vi "Denoise - 1D Real Signal.vi"() -> ()   [LabVIEW 2023]
doc: "This example shows different denoising performances of the methods based on the discrete wavelet transform (DWT) and the undecimated wavelet transform (UWT). The UWT-based method can reduce the Gibbs oscillation effectively from a signal. The denoising result of the UWT-based method is smoother. But the UWT-based method needs more computation time than the DWT-based method. If the computational complexity is limited, you can use the DWT-based method as a compromise. The WA Denoise VI provides both the DWT-based method and the UWT-based method.\n\n<b>Instructions:</b>\n1) Run this VI.\n2) Compare the denoising performance of DWT-based and UWT-based methods with different settings."
uses:
  <vilib>/addons/Wavelet Analysis/typedefs.llb/WA Data.ctl
  <vilib>/addons/Wavelet Analysis/application.llb/WA Denoise (UWT Waveform).vi
  <vilib>/addons/Wavelet Analysis/application.llb/WA Denoise (DWT Waveform).vi
  <vilib>/addons/_Advanced Signal Processing/NI_AdvSigProcWA.lvlib
panel:
  in  "Option for Approx Coef":u16(ring) items=["None", "Threshold", "Detrend"]
  in  "stop":bool
  in  "Threshold settings":T1={"Thresholding Rule"=enum."Minimax", "Rescaling Method"=enum."Single level", "Soft Threshold?"=TRUE}
  out "Denoised Signals":waveform(dbl)[](graph)
  out "Signal":waveform(dbl)(graph)
  in  "Levels":i32=5
  in  "Wavelet":u16(ring) items=["db02"=0, "db03"=1, "db04"=2, "db05"=3, "db06"=4, "db07"=5, "db08"=6, "db09"=7, "db10"=8, "db11"=9, "db12"=10, "db13"=11, "db14"=12, "Haar"=13, "bior1_3"=14, "bior1_5"=15, "bior2_2"=16, "bior2_4"=17, "bior2_6"=18, "bior2_8"=19, "bior3_1"=20, "bior3_3"=21, "bior3_5"=22, "bior3_7"=23, "bior3_9"=24, "bior4_4 (FBI)"=25, "bior5_5"=38, "bior6_8"=39, "coif1"=26, "coif2"=27, "coif3"=28, "coif4"=29, "coif5"=30, "sym2"=31, "sym3"=32, "sym4"=33, "sym5"=34, "sym6"=35, "sym7"=36, "sym8"=37]
  # "Overview: Shows different denoising performances of the methods based on the discrete wavelet transform (DWT) and the undecimated wavelet transform (UWT). \nRequirements: LabVIEW Full Development System, Advanced Signal Processing Toolkit\nInstructions: \n1. Run this VI.\n2. Compare the denoising performance of DWT-based and UWT-based methods with different settings.\n3. Click Stop to stop the VI."
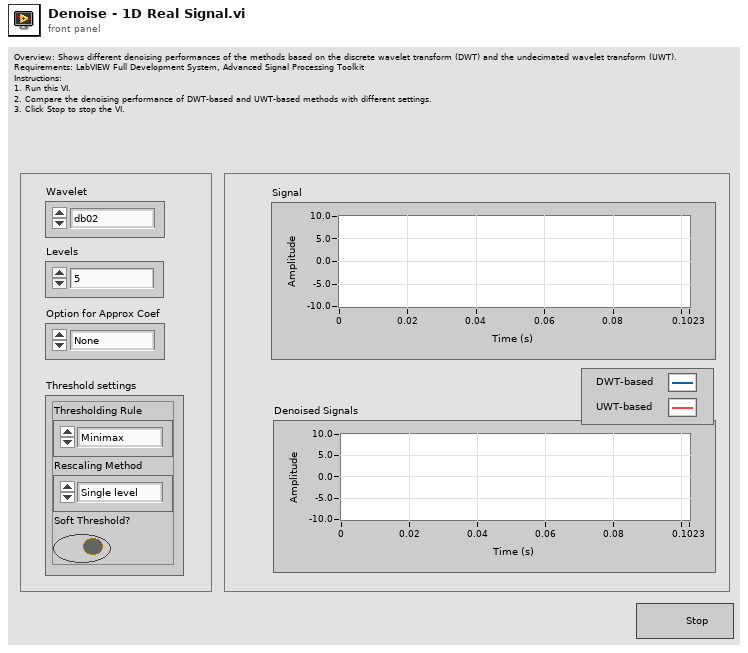
[diagram p1: front panel]
types:
  T1 = cluster{"Thresholding Rule":enum16{"SURE", "Hybrid", "Universal", "Minimax"}, "Rescaling Method":enum16{"One", "Single level", "Multiple levels"}, "Soft Threshold?":bool}
  T2 = typedef "NI_AdvSigProcWA.lvlib/WA Data.ctl" = u16
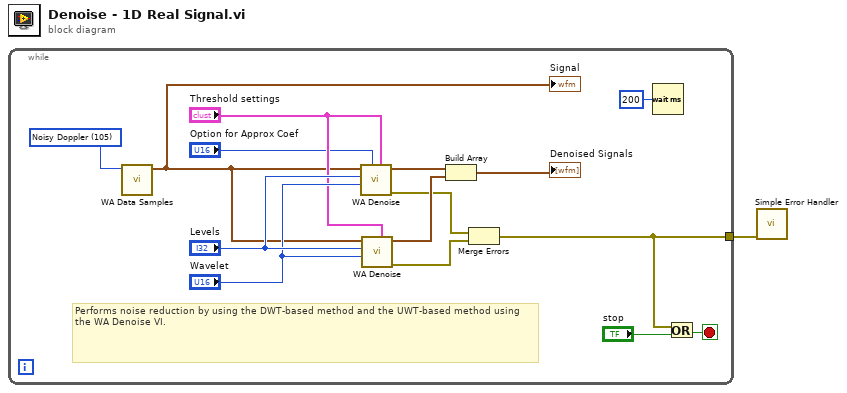
[diagram p0: block diagram]
diagram:
  n1 = while {
    tunnel: [w2] -> w1
    stop <- w6 stop-if-true
    w4 = T2 105 items=["1D Example Data"=100, "-"=101, "Doppler"=102, "HOP"=103, "TF Sine"=104, "Noisy Doppler"=105, "Sea Temperature"=106, "Sp500"=107, "Power Line"=108, "Engine Knocking"=109, "HeaviSine"=110, "Bumps"=111, "Blocks"=112, "Piece Regular"=113, "HypChirps"=114, "LinChirps"=115, "Chirps"=116, "Piece Polynomial"=117, "ECG"=131, "-"=118, "2D Example Data"=119, "-"=120, "Finger Print (Image)"=121, "Iris Flower (Image)"=122, "Mammogram (Image)"=123, "Lake (Image)"=127, "Two Can 1 (Image)"=132, "Two Can 2 (Image)"=133, "Camera Man (Image)"=134] ("data")
    # "Performs noise reduction by using the DWT-based method and the UWT-based method using the WA Denoise VI."
    n2 = call <vilib>:"WA Data Samples.vi"("data"=w4) -> ("signal"=w11:waveform(dbl))  [unwired: 10 out]
    "Signal" <- w11
    n3 = call-poly <vilib>:"WA Denoise.vi"("threshold settings"="Threshold settings", "option for approx coef"="Option for Approx Coef", "wavelet"="Wavelet", "levels"="Levels", "signal"=w11) -> ("error out"=w9:errorcluster, "denoised signal"=w13:waveform(dbl))  [unwired: 1 in, 4 out]
    n4 = call-poly <vilib>:"WA Denoise.vi"("threshold settings"="Threshold settings", "wavelet"="Wavelet", "levels"="Levels", "signal"=w11) -> ("error out"=w8:errorcluster, "denoised signal"=w10:waveform(dbl))  [unwired: 4 in, 2 out]
    n5 = Build Array(w13, w10) -> (→"Denoised Signals":waveform(dbl)[])
    n6 = Merge Errors(w9, w8) -> (w2:errorcluster)
    n7 = Wait (ms)(milliseconds to wait=u32 200 ("millisecond multiple")) -> ()  [unwired: 1 out]
    n8 = Or(x=w2, y="stop") -> (x .or. y?=w6:bool)
  }
  n9 = call <vilib>:"Simple Error Handler.vi"("error in (no error)"=w1) -> ()  [unwired: 1 in, 8 out]
